vi "UDP3GLOB.vi"() -> ()   [LabVIEW 2009]
uses:
  UDP 3.ctl
panel:
  out "INS Heartbeat":bool
  out "UDP Heartbeat":bool
  out "GPS Main Loop Timer (ms)":u32=1
  out "GPS Heartbeat":bool
  in  "stop":bool
  in  "UDP 3":T1
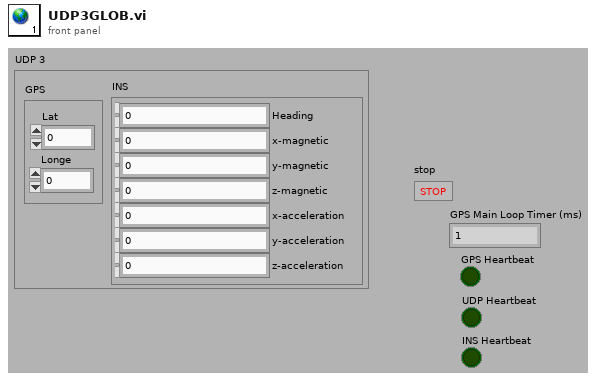
[diagram p1: front panel]
types:
  T1 = typedef "UDP 3.ctl" = cluster{"GPS":cluster{"Lat":dbl, "Longe":dbl}, "INS":cluster{"Heading":dbl, "x-magnetic":dbl, "y-magnetic":dbl, "z-magnetic":dbl, "x-acceleration":dbl, "y-acceleration":dbl, "z-acceleration":dbl}}
diagram:
